vi "Add_Pressure_Cube_Positions.vi"() -> (5 "Plug in titles":string[](array[string]), 7 "Plug in values":string[](array[string]))   [LabVIEW 2016]
uses:
  Globals/Meas_global.vi
panel:
  out "number":i32[][](array[numeric])
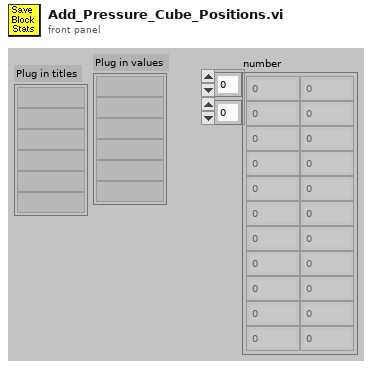
[diagram p1: front panel]
types:
  T1 = typedef "Post_Process.ctl" = enum16{"Take New Data", "Post Process Raw Data File"}
  T2 = typedef "Ch_and_Spans.ctl" = cluster{"high limit (10V)":sgl, "low limit (-10V)":sgl, "Ch No":i16, "Var name":string, "Use Latest Calib":bool}
  T3 = typedef "Analysis_info_cluster.ctl" = cluster{"Colour":u32, "Inst type":T4, "Inst name":string, "Symbol":string, "Code name":string, "Extra Info":string, "Inst Array":T5, "Extra Titles":string[], "Extra Values":string[], "U":dbl, "u^2":dbl, "u^3":dbl, "u^4":dbl, "Skew_u":dbl, "Kurt_u":dbl, "Sd Error in Mean":dbl, "% u'/U":dbl, "X":dbl, "Y":dbl, "Z":dbl, "Timescale integral to 25%":dbl, "Sd Error in Variance":dbl, "Calib File":path, "Calib Constants":dbl[], "Output Position":bool, "Full Stats":bool, "Av Sampling Rate":dbl, "Av No of Samples":dbl, "Total Meas Time (s)":dbl, "ADAM Ch Name":string, "Max value":dbl, "Min value":dbl}
  T4 = typedef "Inst_type.ctl" = enum16{"Propeller anemometer", "Raw voltage", "Pressure Transducer", "Pitot-static tube", "Preston tube", "Hot wire", "Cross wire 1", "Cross wire 2", "Generic Linear", "Generic Polynomial", "Generic BackPoly", "Fast FID", "Thermocouple", "Cold wire", "Pulsed Wire", "LDA Vel", "LDA Tran time", "LDA Arr time", "Microphone"}
  T5 = typedef "Instrument_Array.ctl" = enum16{"PWA", "LDA", "Analogue"}
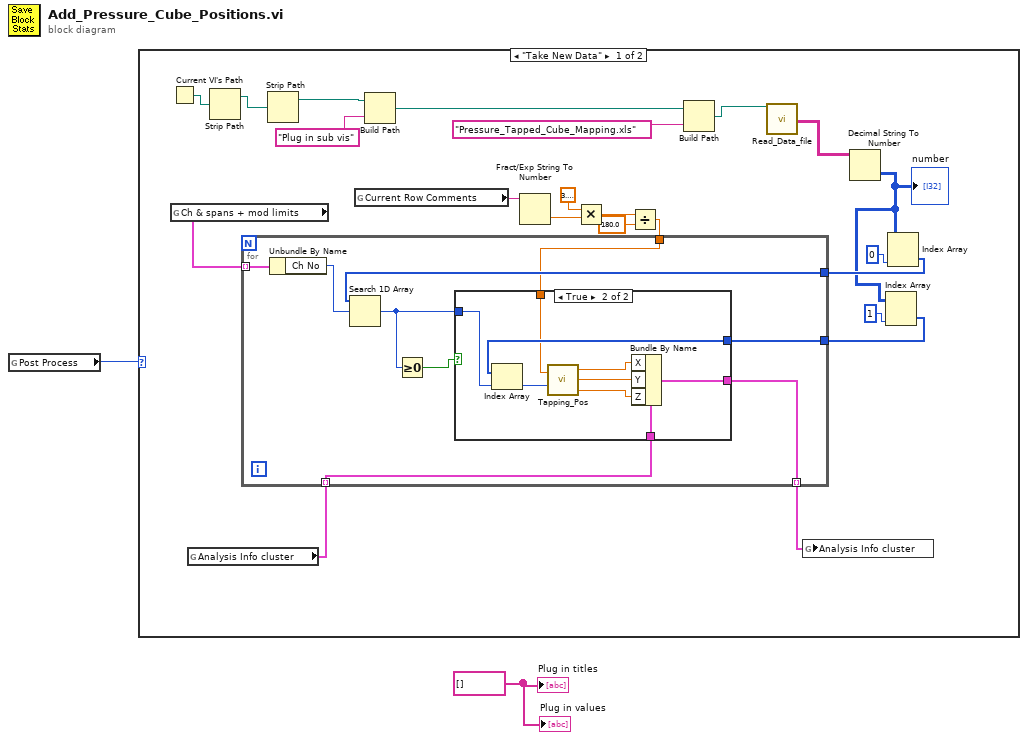
[diagram p0: block diagram]
diagram:
  w2 = string[] [] ("Plug in titles")
  n1 = global read "Meas_global.vi" "Post Process"() -> (w1:T1)
  n2 = case shown="\"Take New Data\"" w1 {
    frame "Take New Data" {
      n3 = Current VI's Path() -> (path=w20:path)
      n4 = global read "Meas_global.vi" "Ch & spans + mod limits"() -> (w24:T2[])
      n5 = global read "Meas_global.vi" "Analysis Info cluster"() -> (w23:T3[])
      n6 = Strip Path(path=w20) -> (stripped path=w19:path)  [unwired: 1 out]
      n7 = Strip Path(path=w19) -> (stripped path=w18:path)  [unwired: 1 out]
      n8 = global read "Meas_global.vi" "Current Row Comments"() -> (w21:string)
      n9 = Build Path(base path=w18, name or relative path="Plug in sub vis") -> (appended path=w16:path)
      n10 = Fract/Exp String To Number(string=w21) -> (number=w7:dbl)  [unwired: 3 in, 1 out]
      n11 = Multiply(x=3.141592653589793, y=w7) -> (x*y=w5:dbl)
      n12 = Divide(x=w5, y=180.0) -> (x/y=w3:dbl)
      n13 = Build Path(base path=w16, name or relative path="Pressure_Tapped_Cube_Mapping.xls") -> (appended path=w14:path)
      n14 = call "Read_Data_file.vi"("Results file"=w14) -> ("Channel Values Out"=w13:string[][])  [unwired: 9 in, 9 out]
      n15 = Decimal String To Number(string=w13) -> (number=w9:i32[][])  [unwired: 2 in, 1 out]
      "number" <- w9
      n16 = Index Array(array=w9, index (col)=1 ("index (row)")) -> (element=w8:i32[])  [unwired: 1 in]
      n17 = Index Array(array=w9, index (col)=0 ("index (row)")) -> (element=w12:i32[])  [unwired: 1 in]
      n18 = for {
        tunnel: w24 -> [w33] mode=indexing
        tunnel: w23 -> [w32] mode=indexing
        tunnel: [w31] -> w22 mode=indexing
        tunnel: w12 -> [w30]
        tunnel: w8 -> [w28]
        tunnel: w3 -> [w25]
        n19 = Unbundle By Name(w33) -> ("Ch No"=w29:i16)
        n20 = Search 1D Array(1D array=w30, element=w29) -> (index of element=w27:i32)  [unwired: 1 in]
        n21 = Greater Or Equal To 0?(x=w27) -> (x >= 0?=w26:bool)
        n22 = case shown="True" w26 {
          tunnel: w32 -> [w34 w43]
          tunnel: [w34 w42] -> w31
          tunnel: w28 -> [_ w38]
          tunnel: w27 -> [_ w36]
          tunnel: w25 -> [_ w35]
          frame False {
          }
          frame True {
            n23 = Index Array(array=w38, index=w36) -> (element=w37:i32)
            n24 = call "Tapping_Pos.vi"("Orientation (rad)"=w35, "Tapping Number"=w37) -> ("X"=w39:sgl, "Y"=w40:sgl, "Z"=w41:sgl)
            n25 = Bundle By Name(cluster=w43, "X"=w39, "Y"=w40, "Z"=w41) -> (w42:T3)
          }
        }
      }
      n26 = global write "Meas_global.vi" "Analysis Info cluster"(w22) -> ()
    }
    frame "Post Process Raw Data File" {
    }
  }
  "Plug in values" <- w2
  "Plug in titles" <- w2
